vi "Read Measurement (Delta Time).vi"(0 "VISA resource name":refnum<visa-resource-name>, 5 "Channel1 (1: Channel 1)":u16(ring)=1 items=["Channel 1"=1, "Channel 2"=2, "Channel 3"=3, "Channel 4"=4, "Function 1"=5, "Function 2"=6, "Function 3"=7, "Function 4"=8, "Memory 1"=9, "Memory 2"=10, "Memory 3"=11, "Memory 4"=12], 7 "Channel2 (2: Channel 2)":u16(ring)=2 items=["Channel 1"=1, "Channel 2"=2, "Channel 3"=3, "Channel 4"=4, "Function 1"=5, "Function 2"=6, "Function 3"=7, "Function 4"=8, "Memory 1"=9, "Memory 2"=10, "Memory 3"=11, "Memory 4"=12], 9 "Maximum Time (10000ms)":u32=10000, 11 "error in (no error)":errorcluster) -> (4 "VISA resource name out":refnum<visa-resource-name>, 6 "Delta Time(s)":dbl, 15 "error out":errorcluster)   [LabVIEW 2012, in "Agilent 8000 Series.lvlib"]
doc: "Measures the delta time between two edges. If one source is specified, the delta time from leading edge of the specified source to the trailing edge of the specified source is measured. If two sources are specified, the delta time from leading edge on the first source to the trailing edge on the second source is measured.\n\nThe start edge and the stop edge of the measured sources are defined by Configure Measurement Characteristics (DeltaTime).vi.\n\nThis VI initiates an acquisition on the channel that the end-user defines. It then waits for the acquisition to complete, obtains a waveform measurement on the channel the end-user specifies, and returns the measurement value."
uses:
  Agilent 8000 Series.lvlib
  Low Level/Fetch Measurement (Delta Time).vi
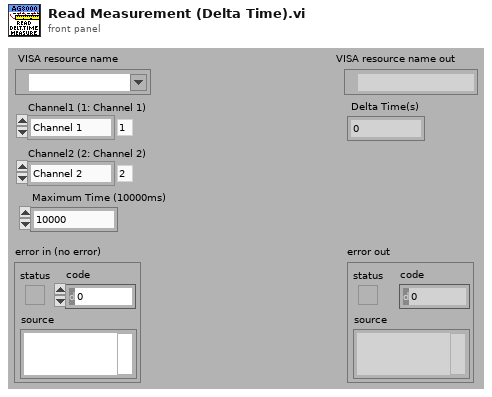
[diagram p1: front panel]
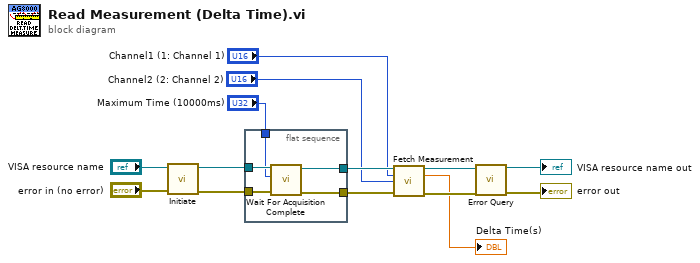
[diagram p0: block diagram]
diagram:
  n1 = call "Initiate.vi"("error in (no error)"="error in (no error)", "VISA resource name"="VISA resource name") -> ("error out"=w9:errorcluster, "VISA resource name out"=w10:refnum<visa-resource-name>)  [unwired: 8 in]
  n2 = flat-sequence {
    tunnel: w10 -> [w19]
    tunnel: w9 -> [w18]
    tunnel: [w17] -> w8
    tunnel: [w16] -> w7
    tunnel: "Maximum Time (10000ms)" -> [w15]
    frame #0 {
      n3 = call "Wait For Acquisition Complete.vi"("error in (no error)"=w18, "Maximum Time (10000ms)"=w15, "VISA resource name"=w19) -> ("error out"=w16:errorcluster, "VISA resource name out"=w17:refnum<visa-resource-name>)  [unwired: 7 in]
    }
  }
  n4 = call-poly "Fetch Measurement.vi"("VISA resource name"=w8, "Channel1 (1: Channel 1)"="Channel1 (1: Channel 1)", "Channel2 (2: Channel 2)"="Channel2 (2: Channel 2)", "error in (no error)"=w7) -> ("VISA resource name out"=w5:refnum<visa-resource-name>, "Delta Time(s)"=→"Delta Time(s)":dbl, "error out"=w6:errorcluster)  [unwired: 9 in]
  n5 = call "Error Query.vi"("error in (no error)"=w6, "VISA resource name"=w5) -> ("error out"=→"error out":errorcluster, "VISA resource name out"=→"VISA resource name out":refnum<visa-resource-name>)  [unwired: 6 in, 2 out]
